vi "Mean.vi"(10 "Array":dbl[](array[numeric])) -> (2 "Mean":dbl)   [LabVIEW 2012]
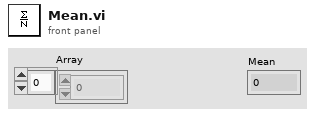
[diagram p1: front panel]
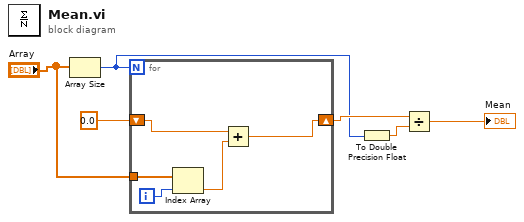
[diagram p0: block diagram]
diagram:
  n1 = Array Size(array="Array") -> (size(s)=w2:i32)
  n2 = for {
    N: w2 -> [_]
    shift-right: [w8] -> w4
    shift-left: 0.0 -> [w9]
    tunnel: "Array" -> [w10]
    i -> [w11]
    n3 = Index Array(array=w10, index=w11) -> (element=w7:dbl)
    n4 = Add(x=w9, y=w7) -> (x+y=w8:dbl)
  }
  n5 = To Double Precision Float(number=w2) -> (double precision float=w3:dbl)
  n6 = Divide(x=w4, y=w3) -> (x/y=→"Mean":dbl)
